vi "Procedure Parameters (A).vi"(0 "LoadProcedure":refnum<k24>, 1 "Command":string(combo), 2 "Command Parameter":string(combo), 3 "EnumSet":i32(ring) items=["Off", "On"], 4 "DoubleSet":dbl, 5 "IntSet":i32, 6 "BoolSet":bool, 8 "SetEnum":bool, 9 "SetDouble":bool, 10 "SetInt":bool, 11 "SetBool":bool, 27 "error in (no error)":errorcluster) -> (7 "error out":errorcluster, 16 "IntGet":i32, 17 "0, 1":i16, 18 "EnumGet":i32(ring) items=["Off", "On"], 19 "DoubleGet":dbl, 20 "Command Names":string[](array[string]), 21 "Command Parameters":string[](array[string]), 22 "VisibleEnum":bool, 23 "VisibleInt":bool, 24 "VisibleDouble":bool, 25 "VisableBool":bool)   [LabVIEW 2011]
doc: "Changes the procedure parameters manually. First select Command then the Command Parameter (advanced version)."
uses:
  C:/Program Files/Metrohm Autolab/Autolab SDK 1.10/EcoChemie.Autolab.Sdk.dll
  EcoChemie.Autolab.Sdk.dll
  C:/Program Files/Metrohm Autolab/Autolab SDK 1.10/EcoChemie100.dll
  EcoChemie100.dll
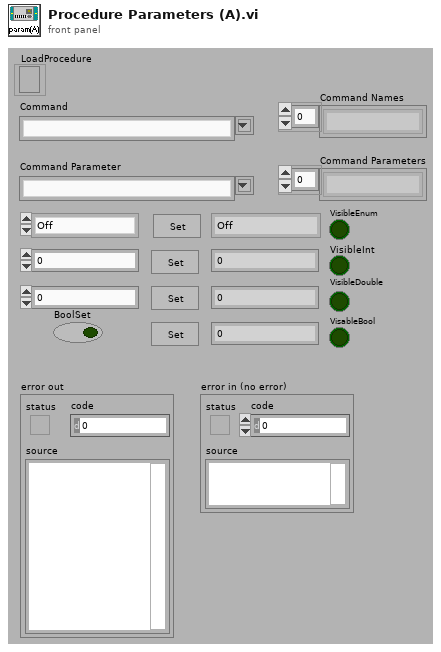
[diagram p1: front panel]
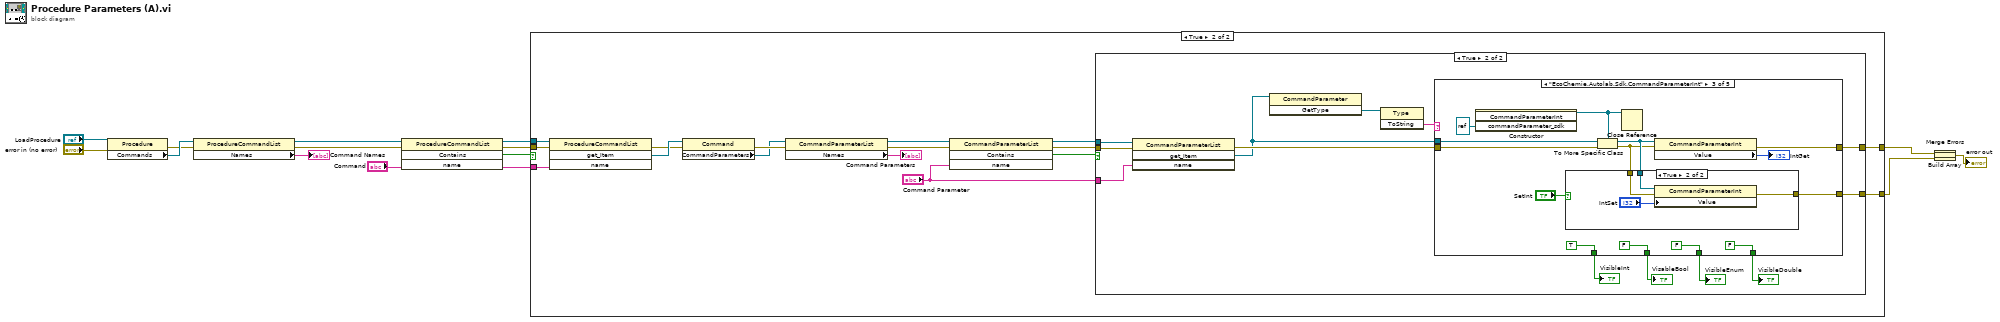
[diagram p0: block diagram]
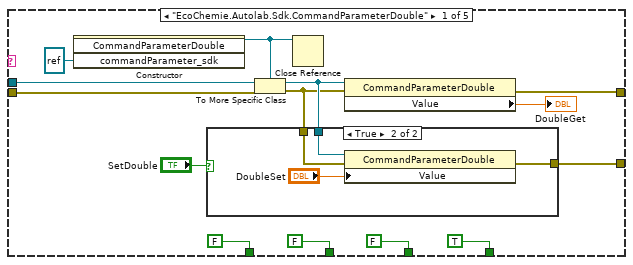
[diagram p4: hidden frame]
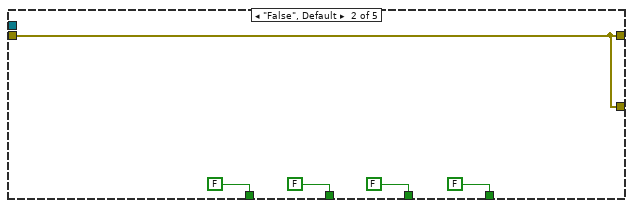
[diagram p6: hidden frame]
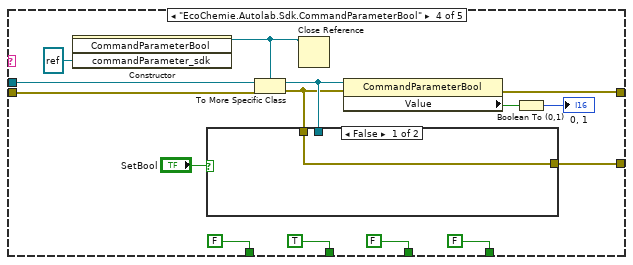
[diagram p8: hidden frame]
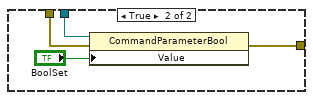
[diagram p9: hidden frame]
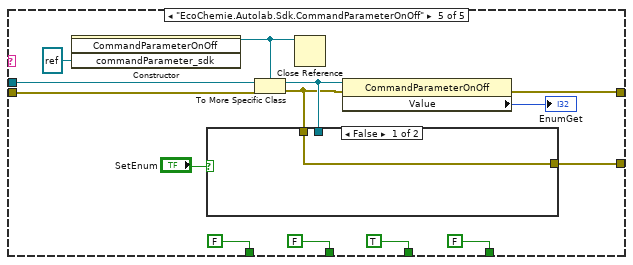
[diagram p10: hidden frame]
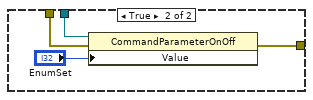
[diagram p11: hidden frame]
diagram:
  n1 = property class="Procedure"(reference="LoadProcedure", error in="error in (no error)") -> (error out=w14:errorcluster, "Commands"=w15:refnum<k24>)  [unwired: 1 out]
  n2 = property class="ProcedureCommandList"(reference=w15, error in=w14) -> (reference out=w13:refnum<k24>, error out=w12:errorcluster, "Names"=→"Command Names":string[])
  n3 = invoke class="ProcedureCommandList" method="Contains"(reference=w13, error in=w12, "name"="Command") -> (reference out=w9:refnum<k24>, error out=w8:errorcluster, "Contains"=w7:bool)  [unwired: 1 in, 1 out]
  n4 = case shown="True" w7 {
    tunnel: w9 -> [_ w32]
    tunnel: w8 -> [w16 w31]
    tunnel: "Command" -> [_ w28]
    tunnel: [w16 w18] -> w5
    tunnel: [w16 w17] -> w4
    frame False {
    }
    frame True {
      n5 = invoke class="ProcedureCommandList" method="get_Item"(reference=w32, error in=w31, "name"=w28) -> (error out=w29:errorcluster, "get_Item"=w30:refnum<k24>)  [unwired: 1 in, 2 out]
      n6 = property class="Command"(reference=w30, error in=w29) -> (error out=w27:errorcluster, "CommandParameters"=w24:refnum<k24>)  [unwired: 1 out]
      n7 = property class="CommandParameterList"(reference=w24, error in=w27) -> (reference out=w26:refnum<k24>, error out=w25:errorcluster, "Names"=→"Command Parameters":string[])
      n8 = invoke class="CommandParameterList" method="Contains"(reference=w26, error in=w25, "name"="Command Parameter") -> (reference out=w20:refnum<k24>, error out=w21:errorcluster, "Contains"=w19:bool)  [unwired: 1 in, 1 out]
      n9 = case shown="True" w19 {
        tunnel: w20 -> [_ w46]
        tunnel: "Command Parameter" -> [_ w43]
        tunnel: w21 -> [w33 w45]
        tunnel: [w33 w38] -> w18
        tunnel: [w33 w37] -> w17
        frame False {
        }
        frame True {
          n10 = invoke class="CommandParameterList" method="get_Item"(reference=w46, error in=w45, "name"=w43) -> (error out=w44:errorcluster, "get_Item"=w35:refnum<k24>)  [unwired: 1 in, 2 out]
          n11 = invoke class="CommandParameter" method="GetType"(reference=w35) -> ("GetType"=w36:refnum<k24>)  [unwired: 2 in, 2 out]
          n12 = invoke class="Type" method="ToString"(reference=w36) -> ("ToString"=w34:string)  [unwired: 2 in, 2 out]
          n13 = case shown="\"EcoChemie.Autolab.Sdk.CommandParameterInt\"" w34 {
            tunnel: w35 -> [w56 _ w79 w99 w118]
            tunnel: w44 -> [w54 w66 w78 w98 w116]
            tunnel: [FALSE FALSE TRUE FALSE FALSE] -> w39
            tunnel: [FALSE FALSE FALSE TRUE FALSE] -> w42
            tunnel: [FALSE FALSE FALSE FALSE TRUE] -> w41
            tunnel: [TRUE FALSE FALSE FALSE FALSE] -> w40
            tunnel: [w50 w66 w74 w94 w113] -> w38
            tunnel: [w49 w66 w73 w93 w112] -> w37
            frame "EcoChemie.Autolab.Sdk.CommandParameterDouble" {
              n14 = constructor class="CommandParameterDouble"("commandParameter_sdk"=refnum<k24> refnum) -> (reference out=w48:refnum<k24>)  [unwired: 3 in, 3 out]
              n15 = To More Specific Class(target class=w48, reference=w56, error in=w54) -> (specific class reference=w55:refnum<k24>, error out=w53:errorcluster)
              n16 = case shown="True" "SetDouble" {
                tunnel: w55 -> [_ w65]
                tunnel: w53 -> [w61 w64]
                tunnel: [w61 w62] -> w49
                frame False {
                }
                frame True {
                  n17 = property class="CommandParameterDouble"(reference=w65, error in=w64, "Value"="DoubleSet") -> (error out=w62:errorcluster)  [unwired: 1 out]
                }
              }
              n18 = Close Reference(reference=w48) -> ()  [unwired: 1 in, 1 out]
              n19 = property class="CommandParameterDouble"(reference=w55, error in=w53) -> (error out=w50:errorcluster, "Value"=→"DoubleGet":dbl)  [unwired: 1 out]
            }
            frame "False", Default {
            }
            frame "EcoChemie.Autolab.Sdk.CommandParameterInt" {
              n20 = constructor class="CommandParameterInt"("commandParameter_sdk"=refnum<k24> refnum) -> (reference out=w72:refnum<k24>)  [unwired: 3 in, 3 out]
              n21 = To More Specific Class(target class=w72, reference=w79, error in=w78) -> (specific class reference=w80:refnum<k24>, error out=w77:errorcluster)
              n22 = case shown="True" "SetInt" {
                tunnel: w80 -> [_ w89]
                tunnel: w77 -> [w85 w88]
                tunnel: [w85 w86] -> w73
                frame False {
                }
                frame True {
                  n23 = property class="CommandParameterInt"(reference=w89, error in=w88, "Value"="IntSet") -> (error out=w86:errorcluster)  [unwired: 1 out]
                }
              }
              n24 = Close Reference(reference=w72) -> ()  [unwired: 1 in, 1 out]
              n25 = property class="CommandParameterInt"(reference=w80, error in=w77) -> (error out=w74:errorcluster, "Value"=→"IntGet":i32)  [unwired: 1 out]
            }
            frame "EcoChemie.Autolab.Sdk.CommandParameterBool" {
              n26 = constructor class="CommandParameterBool"("commandParameter_sdk"=refnum<k24> refnum) -> (reference out=w91:refnum<k24>)  [unwired: 3 in, 3 out]
              n27 = To More Specific Class(target class=w91, reference=w99, error in=w98) -> (specific class reference=w100:refnum<k24>, error out=w92:errorcluster)
              n28 = case shown="False" "SetBool" {
                tunnel: w100 -> [_ w109]
                tunnel: w92 -> [w105 w108]
                tunnel: [w105 w106] -> w93
                frame False {
                }
                frame True {
                  n29 = property class="CommandParameterBool"(reference=w109, error in=w108, "Value"="BoolSet") -> (error out=w106:errorcluster)  [unwired: 1 out]
                }
              }
              n30 = Close Reference(reference=w91) -> ()  [unwired: 1 in, 1 out]
              n31 = property class="CommandParameterBool"(reference=w100, error in=w92) -> (error out=w94:errorcluster, "Value"=w96:bool)  [unwired: 1 out]
              n32 = Boolean To (0,1)(Boolean=w96) -> (0, 1=→"0, 1":i16)
            }
            frame "EcoChemie.Autolab.Sdk.CommandParameterOnOff" {
              n33 = constructor class="CommandParameterOnOff"("commandParameter_sdk"=refnum<k24> refnum) -> (reference out=w111:refnum<k24>)  [unwired: 3 in, 3 out]
              n34 = To More Specific Class(target class=w111, reference=w118, error in=w116) -> (specific class reference=w119:refnum<k24>, error out=w117:errorcluster)
              n35 = case shown="False" "SetEnum" {
                tunnel: w119 -> [_ w128]
                tunnel: w117 -> [w124 w127]
                tunnel: [w124 w125] -> w112
                frame False {
                }
                frame True {
                  n36 = property class="CommandParameterOnOff"(reference=w128, error in=w127, "Value"="EnumSet") -> (error out=w125:errorcluster)  [unwired: 1 out]
                }
              }
              n37 = Close Reference(reference=w111) -> ()  [unwired: 1 in, 1 out]
              n38 = property class="CommandParameterOnOff"(reference=w119, error in=w117) -> (error out=w113:errorcluster, "Value"=→"EnumGet":i32)  [unwired: 1 out]
            }
          }
          "VisableBool" <- w42
          "VisibleEnum" <- w41
          "VisibleDouble" <- w40
          "VisibleInt" <- w39
        }
      }
    }
  }
  n39 = Build Array(w5, w4) -> (w1:errorcluster[])
  n40 = Merge Errors(w1) -> (→"error out":errorcluster)
